vi "Read Temperatures Array WAV.vi"(8 "error in":errorcluster, 10 "Source":string, 11 "DAQmx Thermocouple Continuous Read Strategy in":refnum<class "DAQmx Thermocouple Continuous Read Strategy.lvclass">) -> (0 "error out":errorcluster, 2 "Temperatures":waveform(dbl)[](array[waveform]), 3 "DAQmx Thermocouple Continuous Read Strategy out":refnum<class "DAQmx Thermocouple Continuous Read Strategy.lvclass">)   [LabVIEW 2024, in "DAQmx Thermocouple Continuous Read Strategy.lvclass"]
uses:
  DAQmx Thermocouple Continuous Read Strategy.lvclass
  D:/git/HAL/HAL-Devices/Source/Configure Strategies/DAQmx/DAQmx Base Configure Strategy/DAQmx Base Configure Strategy.lvclass
  DAQmx Base Configure Strategy/DAQmx Base Configure Strategy.lvclass/DAQmx Base Configure Strategy.ctl
  DAQmx Base Configure Strategy/DAQmx Base Configure Strategy.lvclass
  <vilib>/DAQmx/read.llb/DAQmx Read (Analog 1D Wfm NChan NSamp).vi
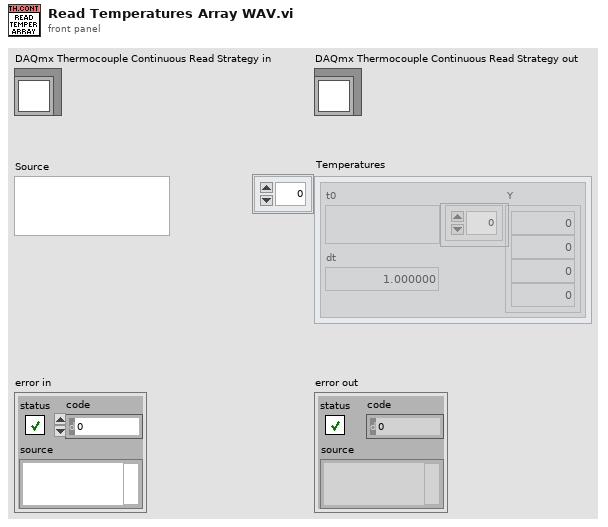
[diagram p1: front panel]
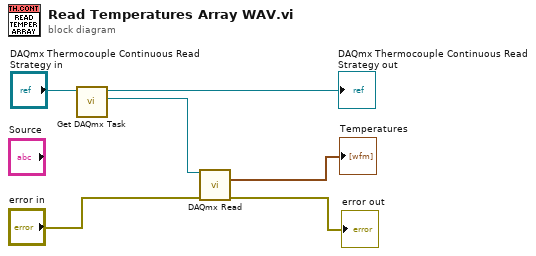
[diagram p0: block diagram]
diagram:
  n1 = call "Get DAQmx Task.vi"("DAQmx Base Configure Strategy in"="DAQmx Thermocouple Continuous Read Strategy in") -> ("DAQmx Task"=w4:refnum<k21>, "DAQmx Base Configure Strategy out"=→"DAQmx Thermocouple Continuous Read Strategy out":refnum<class "DAQmx Thermocouple Continuous Read Strategy.lvclass">)  [unwired: 9 in]
  n2 = call-poly <vilib>:"DAQmx Read.vi"("task/channels in"=w4, "error in"="error in") -> ("data"=→"Temperatures":waveform(dbl)[], "error out"=→"error out":errorcluster)  [unwired: 11 in, 1 out]
